vi "FRCts20_Backend_INI_Set_Variables.vi"() -> ()   [LabVIEW 2013, in "FRCts20_Backend_Engine.lvlib" / "FRCts20_Backend_INI Controller.lvclass"]
uses:
  FRCts20_Backend_INI Controller.lvclass
  FRCts20_Backend_INI_Revision.ctl
  FRCts20_Backend_Engine.lvlib
panel:
  in  "Notify List":string
  in  "Competition":string
  in  "Stop Button":bool
  in  "Connection String":string="Driver={MySQL ODBC 5.1 Driver};Server=ae-assigner;Database=parkway;User=root; Password=password;Option=3;"
  in  "debug?":bool
  in  "Revision":T1
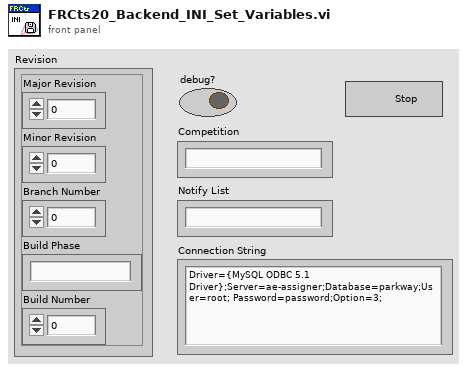
[diagram p1: front panel]
types:
  T1 = typedef "FRCts20_Backend_Engine.lvlib/FRCts20_Backend_INI Controller.lvclass/FRCts20_Backend_INI_Revision.ctl" = cluster{"Major Revision":i32, "Minor Revision":i32, "Branch Number":i32, "Build Phase":string, "Build Number":i32}
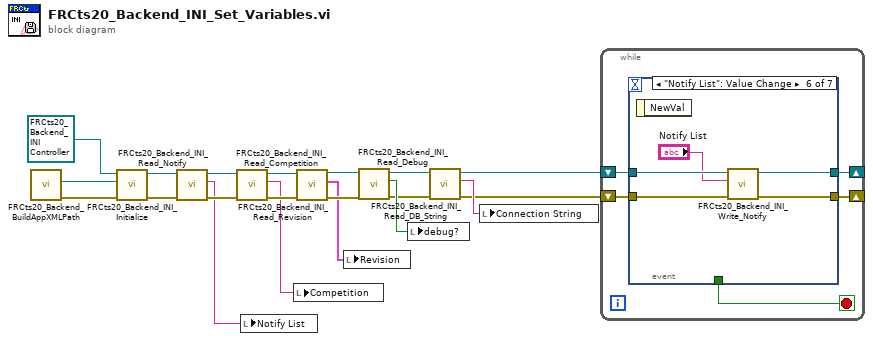
[diagram p0: block diagram]
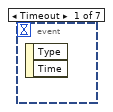
[diagram p2: hidden frame]
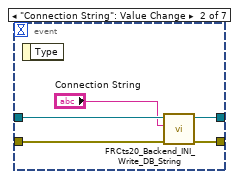
[diagram p3: hidden frame]
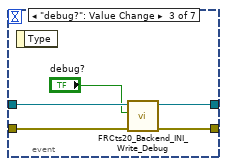
[diagram p4: hidden frame]
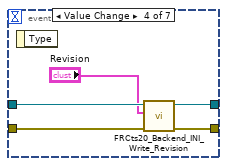
[diagram p5: hidden frame]
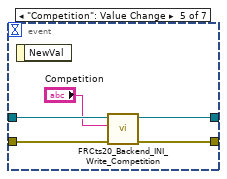
[diagram p6: hidden frame]
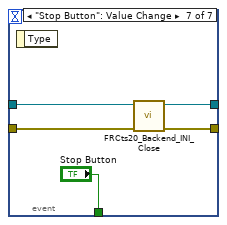
[diagram p7: hidden frame]
diagram:
  n1 = call "FRCts20_Backend_BuildAppXMLPath.vi"() -> ("error out"=w19:errorcluster, "Path Out"=w18:path)  [unwired: 10 in]
  n2 = call "FRCts20_Backend_INI_Initialize.vi"("error in (no error)"=w19, "Config Path"=w18, "INI Controller in"=refnum<class "FRCts20_Backend_INI Controller.lvclass"> refnum ("FRCts20_Backend_Engine.lvlib:INI Controller.lvclass")) -> ("error out"=w5:errorcluster, "INI Controller out"=w4:refnum<class "FRCts20_Backend_INI Controller.lvclass">)  [unwired: 7 in]
  n3 = call "FRCts20_Backend_INI_Read_Notify.vi"("error in (no error)"=w5, "INI Controller in"=w4) -> ("error out"=w2:errorcluster, "Notify List"=w1:string, "INI Controller out"=w3:refnum<class "FRCts20_Backend_INI Controller.lvclass">)  [unwired: 7 in]
  n4 = call "FRCts20_Backend_INI_Read_Competition.vi"("error in (no error)"=w2, "INI Controller in"=w3) -> ("error out"=w7:errorcluster, "Competition Name"=w6:string, "INI Controller out"=w8:refnum<class "FRCts20_Backend_INI Controller.lvclass">)  [unwired: 7 in]
  n5 = local write "Notify List"(w1) -> ()
  n6 = local write "Competition"(w6) -> ()
  n7 = call "FRCts20_Backend_INI_Read_Revision.vi"("error in (no error)"=w7, "INI Controller in"=w8) -> ("error out"=w16:errorcluster, "Revision"=w14:T1, "INI Controller out"=w17:refnum<class "FRCts20_Backend_INI Controller.lvclass">)  [unwired: 7 in]
  n8 = local write "Revision"(w14) -> ()
  n9 = call "FRCts20_Backend_INI_Read_Debug.vi"("error in (no error)"=w16, "INI Controller in"=w17) -> ("error out"=w12:errorcluster, "debug?"=w15:bool, "INI Controller out"=w13:refnum<class "FRCts20_Backend_INI Controller.lvclass">)  [unwired: 7 in]
  n10 = local write "debug?"(w15) -> ()
  n11 = call "FRCts20_Backend_INI_Read_DB_String.vi"("error in (no error)"=w12, "INI Controller in"=w13) -> ("error out"=w9:errorcluster, "Connection String"=w11:string, "INI Controller out"=w10:refnum<class "FRCts20_Backend_INI Controller.lvclass">)  [unwired: 7 in]
  n12 = local write "Connection String"(w11) -> ()
  n13 = while {
    shift-right: [w23] -> _
    shift-left: w10 -> [w25]
    shift-right: [w22] -> _
    shift-left: w9 -> [w24]
    stop <- w21 stop-if-true
    n14 = event shown="[5] \"Notify List\": Value Change" {
      selector: _ -> [_ _ _ _ _ _ _]
      dyn-events: _ -> [_ _ _ _ _ _ _]
      timeout: _ -> [_ _ _ _ _ _ _]
      tunnel: w25 -> [_ w30 w35 w38 w42 w47 w52]
      tunnel: w24 -> [_ w29 w34 w37 w45 w50 w51]
      tunnel: [_ w28 w32 w40 w43 w48 w54] -> w23
      tunnel: [_ w27 w33 w39 w44 w49 w53] -> w22
      tunnel: [_ _ _ _ _ _ "Stop Button"] -> w21
      event Timeout {
        n15 = event-data() -> ()  [unwired: 1 in, 2 out]
      }
      event "Connection String": Value Change {
        n16 = event-data() -> ()  [unwired: 1 in, 1 out]
        n17 = call "FRCts20_Backend_INI_Write_DB_String.vi"("error in (no error)"=w29, "Connection String"="Connection String", "INI Controller in"=w30) -> ("error out"=w27:errorcluster, "INI Controller out"=w28:refnum<class "FRCts20_Backend_INI Controller.lvclass">)  [unwired: 7 in]
      }
      event "debug?": Value Change {
        n18 = event-data() -> ()  [unwired: 1 in, 1 out]
        n19 = call "FRCts20_Backend_INI_Write_Debug.vi"("error in (no error)"=w34, "debug? (F)"="debug?", "INI Controller in"=w35) -> ("error out"=w33:errorcluster, "INI Controller out"=w32:refnum<class "FRCts20_Backend_INI Controller.lvclass">)  [unwired: 7 in]
      }
      event Value Change {
        n20 = event-data() -> ()  [unwired: 1 in, 1 out]
        n21 = call "FRCts20_Backend_INI_Write_Revision.vi"("error in (no error)"=w37, "Revision"="Revision", "INI Controller in"=w38) -> ("error out"=w39:errorcluster, "INI Controller out"=w40:refnum<class "FRCts20_Backend_INI Controller.lvclass">)  [unwired: 7 in]
      }
      event "Competition": Value Change {
        n22 = event-data() -> ()  [unwired: 1 in, 1 out]
        n23 = call "FRCts20_Backend_INI_Write_Competition.vi"("error in (no error)"=w45, "Competition Name"="Competition", "INI Controller in"=w42) -> ("error out"=w44:errorcluster, "INI Controller out"=w43:refnum<class "FRCts20_Backend_INI Controller.lvclass">)  [unwired: 7 in]
      }
      event "Notify List": Value Change {
        n24 = event-data() -> ()  [unwired: 1 in, 1 out]
        n25 = call "FRCts20_Backend_INI_Write_Notify.vi"("error in (no error)"=w50, "Notify List"="Notify List", "INI Controller in"=w47) -> ("error out"=w49:errorcluster, "INI Controller out"=w48:refnum<class "FRCts20_Backend_INI Controller.lvclass">)  [unwired: 7 in]
      }
      event "Stop Button": Value Change {
        n26 = event-data() -> ()  [unwired: 1 in, 1 out]
        n27 = call "FRCts20_Backend_INI_Close.vi"("error in (no error)"=w51, "INI Controller in"=w52) -> ("error out"=w53:errorcluster, "INI Controller out"=w54:refnum<class "FRCts20_Backend_INI Controller.lvclass">)  [unwired: 7 in, 1 out]
      }
    }
  }
